vi "Pie-graphs.vi"(6 "Defect Statistics":refnum<vi>, 7 "Colors":u32[](array[colorbox]), 8 "error in (no error)":errorcluster, 9 "Defect Names":string[](array[string]), 11 "Array Of Values":dbl[](array[numeric])=[0.0, 0.0, 0.0, 0.0, 0.0, 0.0, 0.0]) -> (0 "error out":errorcluster, 1 "Labels":picture, 2 "Report Values":string[][](array[string]), 3 "Pie Graph":picture, 4 "x*y":dbl[](array[numeric]))   [LabVIEW 2015]
uses:
  <vilib>/Utility/miscctls.llb/LVBoundsTypeDef.ctl
  Zen Analytics.lvclass
panel:
  # "Array of collection of No. of passes per month = 1 element\n\nArray of collection of No. of fails per month = 1 element \n\nArray of collection of count of defferent defect values 0\n7 defect values per month\n\nex: DefectFail\n      array values for last 3 months\n      array will have sum of all rows as its separate elements\n      669+669+669\n      669+669+669\n      679+679+679\n      661+661+661\n      665+665+665\n      642+642+642\n      638+638+638"
  # "Defect Names :   Nose gap\n                              Length\n                              Width\n                              Height\n                              Nose width\n                              Nose length\n                              Nose radius"
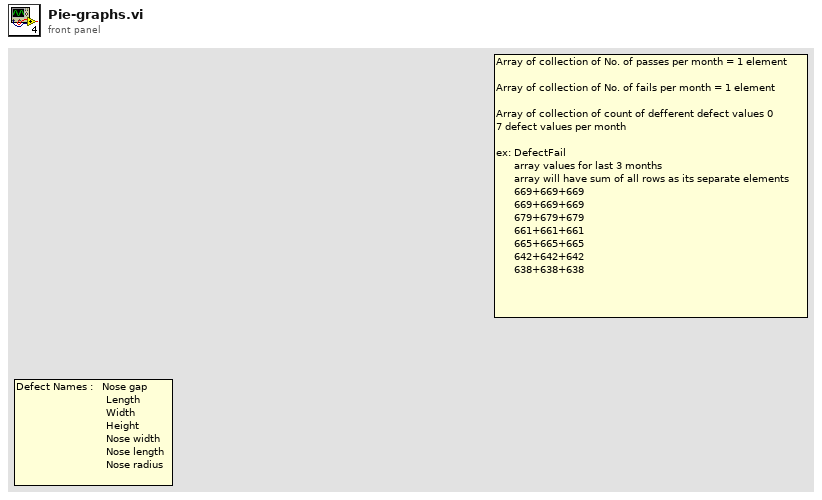
[diagram p1: front panel]
types:
  T1 = typedef "LVBoundsTypeDef.ctl" = cluster{"Width":u32, "Height":u32}
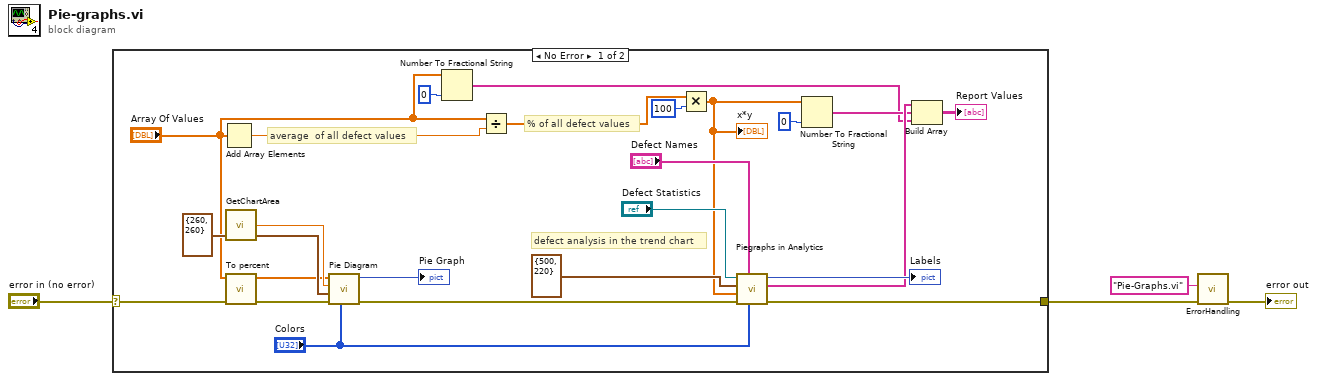
[diagram p0: block diagram]
diagram:
  n1 = case shown="No Error" "error in (no error)" {
    selector: "error in (no error)" -> [w6 w30]
    tunnel: [w5 w30] -> w3
    frame No Error {
      # "defect analysis in the trend chart"
      # "average  of all defect values"
      # "% of all defect values"
      n2 = Add Array Elements(numeric array="Array Of Values") -> (sum=w12:dbl)
      n3 = call "GetChartArea.vi"("Draw Area Size"=T1 {"Width"=260, "Height"=260} ("Draw Area Size 2")) -> ("Chart Area Size"=w26:cluster{"Width":dbl, "Height":dbl}, "Height"=w25:dbl)  [unwired: 3 out]
      n4 = call "To percent.vi"("error in (no error)"=w6, "I/p"="Array Of Values") -> ("error out"=w8:errorcluster, "O/p"=w19:dbl[])  [unwired: 8 in]
      n5 = call "Pie Diagram.vi"("Array"="Colors", "error in (no error)"=w8, "Chart Area Size"=w26, "Height"=w25, "Values"=w19) -> ("error out"=w7:errorcluster, "new picture"=→"Pie Graph":picture)  [unwired: 5 in]
      n6 = Number To Fractional String(number="Array Of Values", precision (6)=i16 0) -> (F-format string=w13:string[])  [unwired: 2 in]
      n7 = Divide(x="Array Of Values", y=w12) -> (x/y=w17:dbl[])
      n8 = Multiply(x=w17, y=100) -> (x*y=w9:dbl[])
      "x*y" <- w9
      n9 = call "Piegraphs in Analytics.vi"("Colors"="Colors", "Defect Names"="Defect Names", "error in (no error)"=w7, "Defect Values"=w9, "Draw Area Size"=T1 {"Width"=500, "Height"=220}, "Defect Statistics"="Defect Statistics") -> ("error out"=w5:errorcluster, "Names with %  values"=w23:string[], "Labels"=→"Labels":picture)  [unwired: 3 in]
      n10 = Number To Fractional String(number=w9, precision (6)=i16 0) -> (F-format string=w18:string[])  [unwired: 2 in]
      n11 = Build Array(w23, w18, w13) -> (→"Report Values":string[][])
    }
    frame Error {
    }
  }
  n12 = call "ErrorHandling.vi"("error in (no error)"=w3, "Vi-name"="Pie-Graphs.vi") -> ("error out"=→"error out":errorcluster)  [unwired: 9 in]
